vi "Test Init Module.vi"(8 "error in (no error)":errorcluster, 11 "TestCase in":refnum<class "Test Osciloscope Init.lvclass">) -> (0 "error out":errorcluster, 3 "TestCase out":refnum<class "Test Osciloscope Init.lvclass">)   [LabVIEW 2020, in "Test Osciloscope Init.lvclass"]
uses:
  Test Osciloscope Init.lvclass
  Libraries/Osciloscope/Osciloscope.lvlib
  <vilib>/addons/_JKI Toolkits/VI Tester/TestCase.llb/TestCase.lvclass
  C:/Program Files (x86)/National Instruments/LabVIEW 2020/vi.lib/addons/_JKI Toolkits/VI Tester/TestCase.llb/TestCase.lvclass
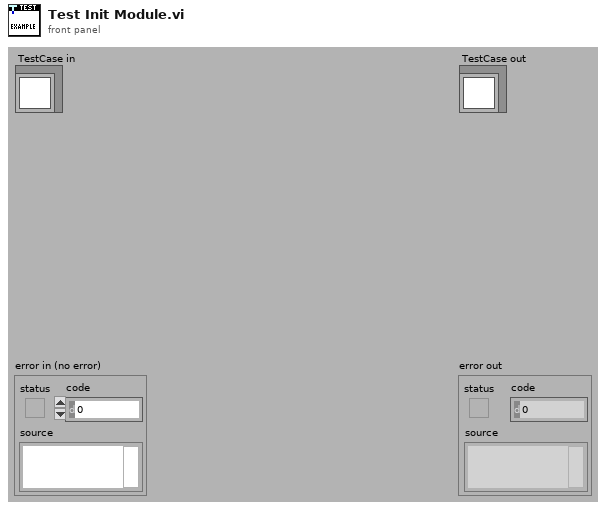
[diagram p1: front panel]
types:
  T1 = typedef "Osciloscope.lvlib/Broadcast Events--cluster.ctl" = cluster{"Module Did Init":refnum<user-event>, "Status Updated":refnum<user-event>, "Error Reported":refnum<user-event>, "Module Did Stop":refnum<user-event>, "Update Module Execution Status":refnum<user-event>, "OsciloscopesTypes":refnum<user-event>}
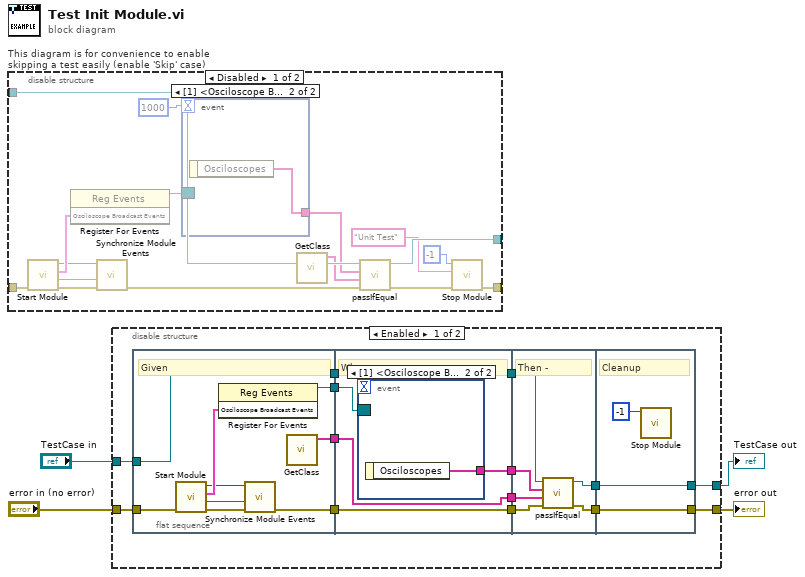
[diagram p0: block diagram]
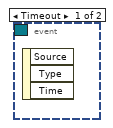
[diagram p2: hidden frame]
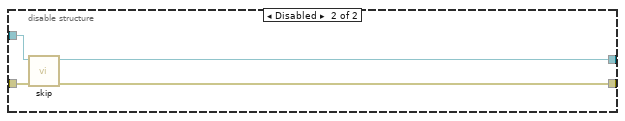
[diagram p3: hidden frame]
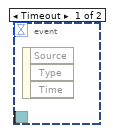
[diagram p4: hidden frame]
diagram:
  n1 = disable-structure "This diagram is for convenience to enable skipping a test easily (enable 'Skip' case)" shown="Disabled" {
    disable-tunnel: _ -> [w20 _]
    disable-tunnel: [w19 _] -> _
    disable-tunnel: [w7 _] -> _
    disable-tunnel: _ -> [w16 _]
    frame Disabled {
      n2 = call "Start Module.vi"("error in"=w16) -> ("error out"=w15:errorcluster, "Wait for Event Sync?"=w18:bool, "Osciloscope Broadcast Events"=w17:T1, "Module ID"=w11:i32)  [unwired: 7 in]
      n3 = register-events(w17) -> (reference out=w14:refnum<event-registration>)  [unwired: 2 in, 1 out]
      n4 = call "Synchronize Module Events.vi"("error in"=w15, "Wait for Event Sync?"=w18, "Module ID in"=w11) -> ("error out"=w9:errorcluster)  [unwired: 7 in, 1 out]
      n5 = event shown="[1] <Osciloscope Broadcast Events.OsciloscopesTypes>: User Event" {
        selector: w14 -> [_ _]
        dyn-events: _ -> [_ _]
        timeout: 1000 -> [_ _]
        tunnel: [_ w21] -> w12
        event Timeout {
          n6 = event-data() -> ()  [unwired: 1 in, 3 out]
        }
        event User Event {
          n7 = event-data() -> ("Osciloscopes"=w21:string[])  [unwired: 1 in]
        }
      }
      n8 = call "GetClass.vi"() -> ("Class Avaliables"=w10:string[])  [unwired: 11 in]
      n9 = call-dynamic "passIfEqual.vi"("error in (no error)"=w9, "y"=w10, "x"=w12, "TestCase in"=w20) -> ("error out"=w8:errorcluster, "TestCase out"=w19:refnum<class "Test Osciloscope Init.lvclass">)  [unwired: 6 in]
      n10 = call "Stop Module.vi"("error in (no error)"=w8, "Origin"="Unit Test", "Module ID"=-1) -> ("error out"=w7:errorcluster)  [unwired: 8 in]
    }
    frame Enabled {
    }
  }
  n11 = disable-structure shown="Enabled" {
    disable-tunnel: [w29 w61] -> w4
    disable-tunnel: [w28 w60] -> w3
    disable-tunnel: "TestCase in" -> [w27 w63]
    disable-tunnel: "error in (no error)" -> [w26 w62]
    frame Enabled {
      n12 = flat-sequence {
        tunnel: w26 -> [w40]
        tunnel: w27 -> [w44]
        tunnel: [w44] -> w35
        tunnel: [w38] -> w34
        tunnel: [w37] -> w25
        tunnel: [w36] -> w22
        tunnel: [w49] -> w33
        tunnel: [w48] -> w32
        tunnel: w35 -> [w49]
        tunnel: w34 -> [w48]
        tunnel: w25 -> [w47]
        tunnel: [w46] -> w24
        tunnel: [w45] -> w23
        tunnel: w22 -> [w45]
        tunnel: [w55] -> w31
        tunnel: [w53] -> w30
        tunnel: w33 -> [w56]
        tunnel: w32 -> [w54]
        tunnel: w24 -> [w52]
        tunnel: w23 -> [w51]
        tunnel: [w58] -> w28
        tunnel: [w59] -> w29
        tunnel: w31 -> [w59]
        tunnel: w30 -> [w58]
        frame #0 {
          # "Given"
          n13 = call "Start Module.vi"("error in"=w40) -> ("error out"=w39:errorcluster, "Wait for Event Sync?"=w43:bool, "Osciloscope Broadcast Events"=w42:T1, "Module ID"=w41:i32)  [unwired: 7 in]
          n14 = register-events(w42) -> (reference out=w37:refnum<event-registration>)  [unwired: 2 in, 1 out]
          n15 = call "Synchronize Module Events.vi"("error in"=w39, "Wait for Event Sync?"=w43, "Module ID in"=w41) -> ("error out"=w38:errorcluster)  [unwired: 7 in, 1 out]
          n16 = call "GetClass.vi"() -> ("Class Avaliables"=w36:string[])  [unwired: 11 in]
        }
        frame #1 {
          # "When -"
          n17 = event shown="[1] <Osciloscope Broadcast Events.OsciloscopesTypes>: User Event" {
            selector: w47 -> [_ _]
            dyn-events: _ -> [_ _]
            timeout: _ -> [_ _]
            tunnel: [_ w50] -> w46
            event Timeout {
              n18 = event-data() -> ()  [unwired: 1 in, 3 out]
            }
            event User Event {
              n19 = event-data() -> ("Osciloscopes"=w50:string[])  [unwired: 1 in]
            }
          }
        }
        frame #2 {
          # "Then -"
          n20 = call-dynamic "passIfEqual.vi"("error in (no error)"=w54, "y"=w51, "x"=w52, "TestCase in"=w56) -> ("error out"=w53:errorcluster, "TestCase out"=w55:refnum<class "Test Osciloscope Init.lvclass">)  [unwired: 6 in]
        }
        frame #3 {
          # "Cleanup"
          n21 = call "Stop Module.vi"("Module ID"=-1) -> ()  [unwired: 10 in, 1 out]
        }
      }
    }
    frame Disabled {
      n22 = call <vilib>:"skip.vi"("error in (no error)"=w62, "TestCase in"=w63) -> ("error out"=w60:errorcluster, "TestCase out"=w61:refnum<class "Test Osciloscope Init.lvclass">)  [unwired: 8 in]
    }
  }
  "error out" <- w3
  "TestCase out" <- w4
